vi "ProjectItemDisplay.vi"(8 "error in (no error)":errorcluster, 11 "Project.lvclass In":refnum<class "Project.lvclass">) -> (0 "error out":errorcluster, 1 "StepNames":string[](array[string]), 2 "ProjectNames":string[](array[string]), 3 "Project.lvclass Out":refnum<class "Project.lvclass">, 4 "VirtualNames":string[](array[string]))   [LabVIEW 2014, in "Project.lvclass"]
uses:
  Project.lvclass
  Project.lvclass/Project.ctl
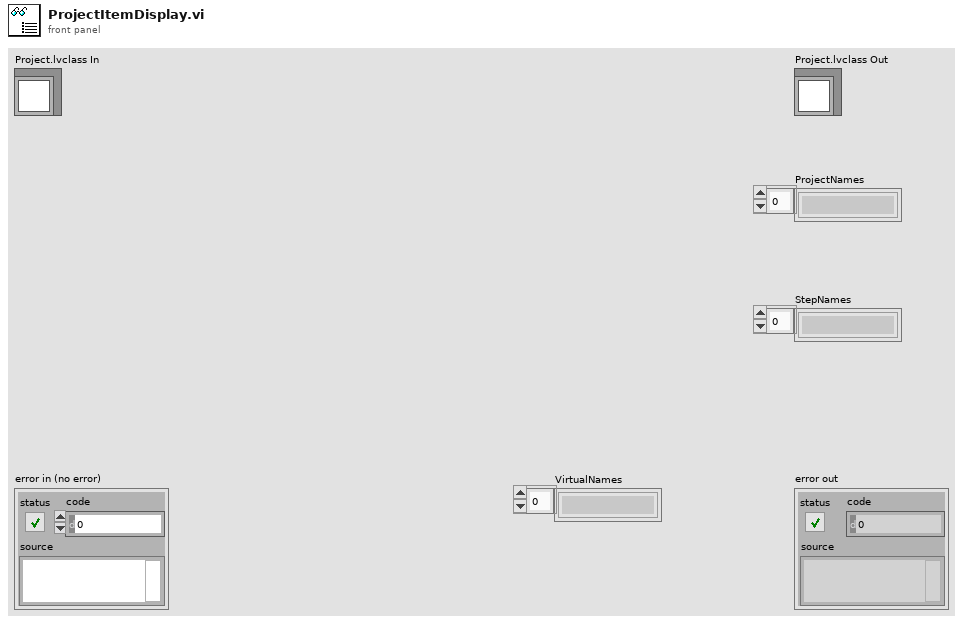
[diagram p1: front panel]
types:
  T1 = typedef "Project.lvclass/ProjectDataTableTypeDefine.ctl" = string[][]
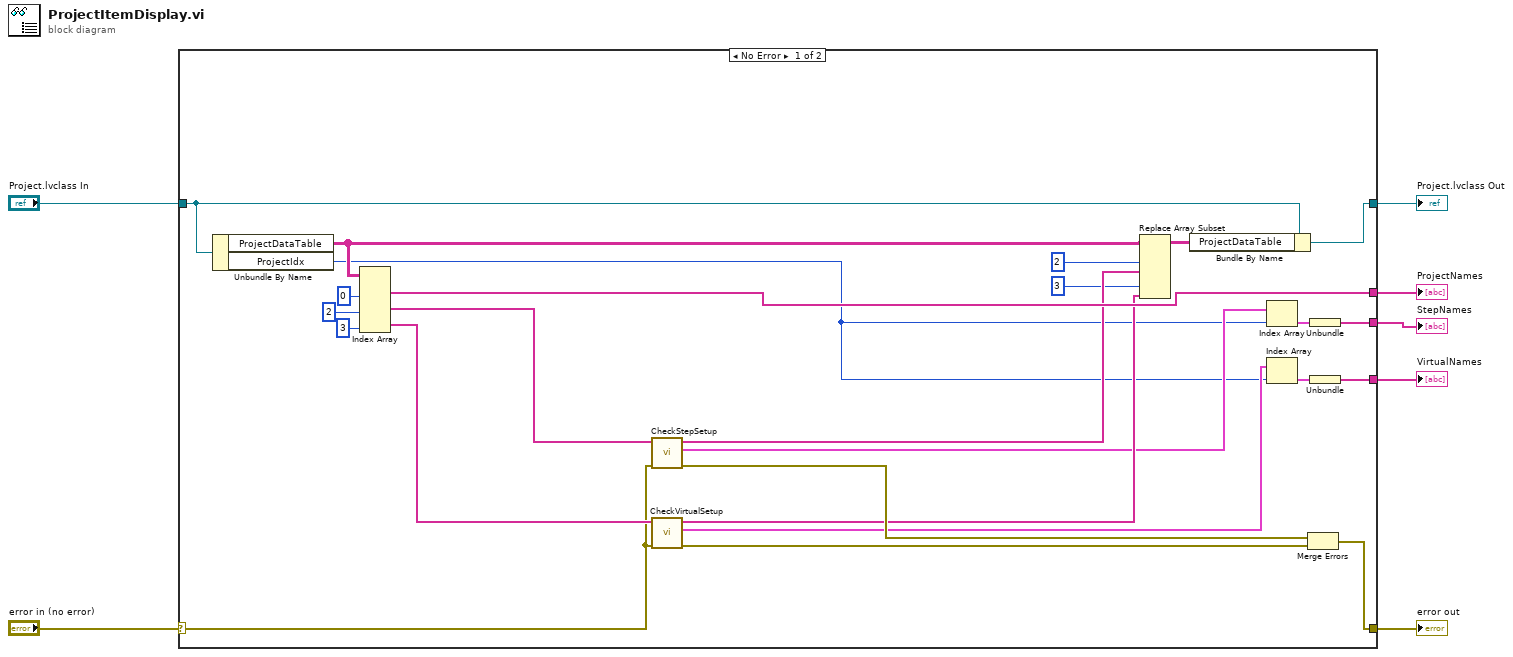
[diagram p0: block diagram]
diagram:
  n1 = case shown="No Error" "error in (no error)" {
    selector: "error in (no error)" -> [w19 w34]
    tunnel: [w16 w34] -> w6
    tunnel: "Project.lvclass In" -> [w31 w33]
    tunnel: [w30 w33] -> w4
    tunnel: [w26 _] -> w3
    tunnel: [w24 _] -> w2
    tunnel: [w9 _] -> w1
    frame No Error {
      n2 = Unbundle By Name(w31) -> ("ProjectDataTable"=w29:T1, "ProjectIdx"=w8:i32)
      n3 = Index Array(array=w29, index (col) #1=0 ("disabled index (col)"), index (col) #2=2 ("index (col)"), index (col) #3=3 ("index (col)")) -> (element #1=w26:string[], element #2=w22:string[], element #3=w20:string[])  [unwired: 3 in]
      n4 = call "CheckStepSetup.vi"("error in (no error)"=w19, "StepDataTable"=w22) -> ("error out"=w18:errorcluster, "StepNames"=w12:cluster{string[]}[], "StepSetups"=w15:string[])  [unwired: 7 in]
      n5 = call "CheckVirtualSetup.vi"("error in (no error)"=w19, "VirtualDataTable"=w20) -> ("error out"=w17:errorcluster, "VirtualNames"=w11:cluster{string[]}[], "VirtualSetups"=w13:string[])  [unwired: 7 in]
      n6 = Replace Array Subset(array=w29, new element #1=w15, index (col) #1=2 ("disabled index (col)"), new element #2=w13, index (col) #2=3 ("index (col)")) -> (w27:T1)  [unwired: 2 in]
      n7 = Bundle By Name(cluster=w31, "ProjectDataTable"=w27) -> (w30:refnum<class "Project.lvclass">)
      n8 = Index Array(array=w12, index=w8) -> (element=w25:cluster{string[]})
      n9 = Index Array(array=w11, index=w8) -> (element=w10:cluster{string[]})
      n10 = Merge Errors(w18, w17) -> (w16:errorcluster)
      n11 = Unbundle(w25) -> (w24:string[])
      n12 = Unbundle(w10) -> (w9:string[])
    }
    frame Error {
    }
  }
  "error out" <- w6
  "Project.lvclass Out" <- w4
  "ProjectNames" <- w3
  "StepNames" <- w2
  "VirtualNames" <- w1
